vi "Observe Data.vi"(6 "Time Stamp":timestamp, 8 "error in (no error)":errorcluster, 9 "Value":variant, 10 "Datum Name":string, 11 "ViewableLEDs in":refnum<class "ViewableLEDs.lvclass">) -> (0 "error out":errorcluster, 3 "ViewableLEDs out":refnum<class "ViewableLEDs.lvclass">)   [LabVIEW 2017, in "ViewableLEDs.lvclass"]
doc: "<License>\nCopyright © 2017 Composed Systems, LLC | All rights reserved\nwww.composed.io\n\nAuthor: Ethan Stern <ethan.stern@composed.io>\n\nThis software is provided \"AS IS\" WITHOUT WARRANTIES, either express or implied, AND IS FOR EDUCATIONAL PURPOSES ONLY.\n</License>MVA Framework 1.7.0.33\nEthan Stern - Composed Systems\nCopyright (c) 2018, Composed Systems"
uses:
  <vilib>/gpm_packages/@cs/example/Dynamic Viewables/ViewableLEDs/ViewableLEDs.lvclass
  <vilib>/gpm_packages/@cs/example/Dynamic Viewables/ViewableLEDs/ViewableLEDs.lvclass/ViewableLEDs.ctl
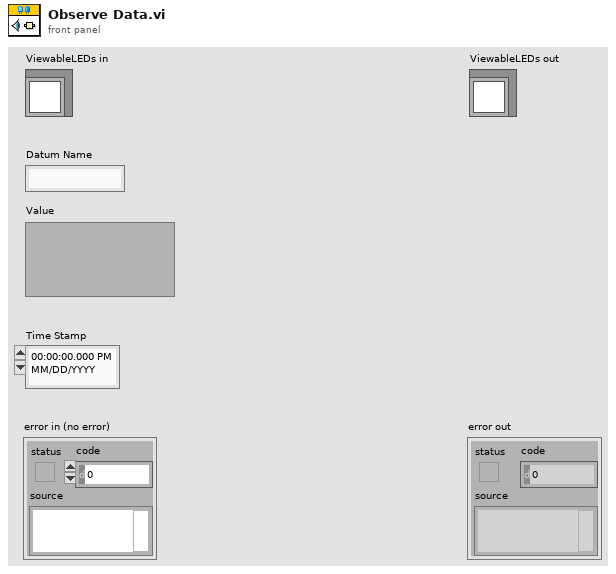
[diagram p1: front panel]
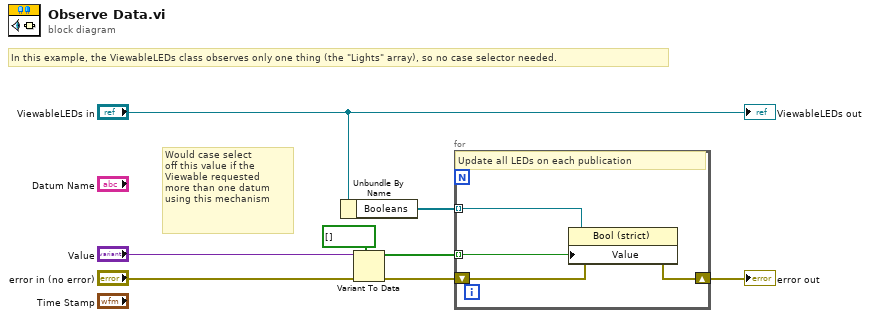
[diagram p0: block diagram]
diagram:
  # "Would case select\noff this value if the\nViewable requested\nmore than one datum\nusing this mechanism"
  # "In this example, the ViewableLEDs class observes only one thing (the \"Lights\" array), so no case selector needed."
  n1 = Unbundle By Name("ViewableLEDs in") -> ("Booleans"=w4:refnum<vi>[])
  n2 = Variant To Data(error in="error in (no error)", type=bool[] [], Variant="Value") -> (data=w3:bool[], error out=w2:errorcluster)
  n3 = for {
    tunnel: w4 -> [w12] mode=indexing
    tunnel: w3 -> [w11] mode=indexing
    shift-right: [w10] -> w1
    shift-left: w2 -> [w9]
    # "Update all LEDs on each publication"
    n4 = property class="Bool (strict)"(reference=w12, error in=w9, "Value"=w11) -> (error out=w10:errorcluster)  [unwired: 1 out]
  }
  "error out" <- w1
  "ViewableLEDs out" <- "ViewableLEDs in"
